vi "VariablesTCShortcutMenuCreate.vi"(8 "error in (no error)":errorcluster, 10 "ShortcutMenuIn":T2, 11 "VMUI in":refnum<class "VMUI.lvclass">) -> (0 "error out":errorcluster, 2 "Discard?":bool, 3 "VMUI out":refnum<class "VMUI.lvclass">)   [LabVIEW 2013, in "VMUI.lvclass"]
uses:
  VMUI.lvclass
  <vilib>/Utility/miscctls.llb/LVPoint32TypeDef.ctl
  VariableManager/VariableManager.lvclass
  VariableGroup/VariableGroup.lvclass
  API/VariableManagerAPI.lvlib
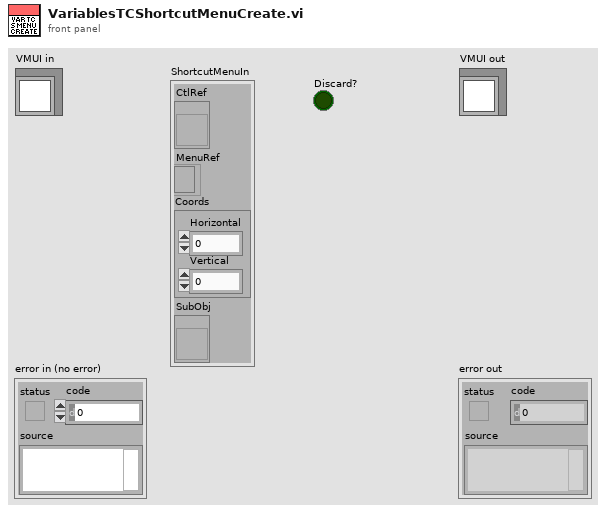
[diagram p1: front panel]
types:
  T1 = typedef "LVPoint32TypeDef.ctl" = cluster{"Horizontal":i32, "Vertical":i32}
  T2 = cluster{"CtlRef":refnum<vi>, "MenuRef":refnum<k9>, "Coords":T1, "SubObj":refnum<vi>}
  T3 = typedef "LVRowAndColumnTypeDef.ctl" = cluster{"Row":i32, "Column":i32}
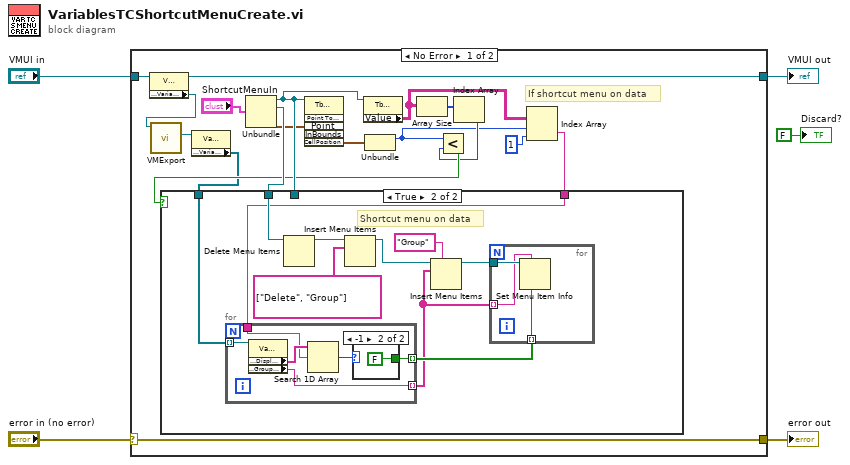
[diagram p0: block diagram]
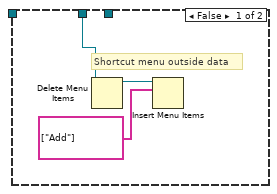
[diagram p2: hidden frame]
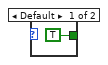
[diagram p3: hidden frame]
diagram:
  n1 = case shown="No Error" "error in (no error)" {
    selector: "error in (no error)" -> [w23 w49]
    tunnel: [w23 w49] -> w4
    tunnel: [w14 w48] -> w2
    tunnel: "VMUI in" -> [w15 w48]
    frame No Error {
      # "If shortcut menu on data"
      n2 = property class="VMUI.lvclass"(reference=w15) -> (reference out=w14:refnum<class "VMUI.lvclass">, "Accessors:VariableManagerRef"=w7:refnum<vi>)  [unwired: 1 in, 1 out]
      n3 = call "VMExport.vi"("VariableManagerRef in"=w7) -> ("VariableManagerExportCopy"=w6:refnum<class "VariableManager.lvclass">)  [unwired: 8 in, 2 out]
      n4 = property class="VariableManager.lvclass"(reference=w6) -> ("Accessors:VariableGroups"=w8:refnum<class "VariableGroup.lvclass">[])  [unwired: 1 in, 2 out]
      n5 = Unbundle("ShortcutMenuIn") -> ("CtlRef"=w22:refnum<vi>, "MenuRef"=w21:refnum<k9>, "Coords"=w16:T1)  [unwired: 1 out]
      n6 = invoke class="Tbl (strict)" method="Point To Row Column"(reference=w22, "Point"=w16) -> ("CellPosition"=w19:T3)  [unwired: 4 in, 5 out]
      n7 = property class="Tbl (strict)"(reference=w22) -> ("Value"=w13:string[][])  [unwired: 1 in, 2 out]
      n8 = Unbundle(w19) -> ("Row"=w12:i32)  [unwired: 1 out]
      n9 = Array Size(array=w13) -> (size(s)=w18:i32[])
      n10 = Index Array(array=w18) -> (element=w17:i32)  [unwired: 1 in]
      n11 = Less?(x=w12, y=w17) -> (x < y?=w20:bool)
      n12 = Index Array(array=w13, index (row)=w12, index (col)=1 ("disabled index (col)")) -> (element=w10:string)
      n13 = case shown="True" w20 {
        tunnel: w21 -> [w26 w35]
        tunnel: w22 -> [_ _]
        tunnel: w8 -> [_ w34]
        tunnel: w10 -> [_ w33]
        frame False {
          # "Shortcut menu outside data"
          n14 = Delete Menu Items(9:w26) -> (3:w25:refnum<k9>)  [unwired: 3 in, 1 out]
          n15 = Insert Menu Items(8:string[] ["Add"] ("item names"), 9:w25) -> ()  [unwired: 4 in, 3 out]
        }
        frame True {
          # "Shortcut menu on data"
          n16 = for {
            tunnel: w34 -> [w45] mode=indexing
            tunnel: w33 -> [w43]
            tunnel: [w41] -> w29 mode=indexing
            tunnel: [w40] -> w28 mode=indexing
            n17 = property class="VariableGroup.lvclass"(reference=w45) -> ("Accessors:DisplayList"=w44:string[], "Accessors:GroupName"=w40:string)  [unwired: 1 in, 2 out]
            n18 = Search 1D Array(1D array=w44, element=w43) -> (index of element=w42:i32)  [unwired: 1 in]
            n19 = case shown="-1" w42 {
              tunnel: [TRUE FALSE] -> w41
              frame Default {
              }
              frame -1 {
              }
            }
          }
          n20 = Delete Menu Items(9:w35) -> (3:w36:refnum<k9>)  [unwired: 3 in, 1 out]
          n21 = Insert Menu Items(8:string[] ["Delete", "Group"] ("item names"), 9:w36) -> (3:w32:refnum<k9>)  [unwired: 4 in, 2 out]
          n22 = Insert Menu Items(5:"Group", 8:w28, 9:w32) -> (3:w30:refnum<k9>)  [unwired: 3 in, 2 out]
          n23 = for {
            tunnel: w30 -> [w39]
            tunnel: w29 -> [w38] mode=indexing
            tunnel: w28 -> [w37] mode=indexing
            n24 = Set Menu Item Info(6:w38, 7:w37, 11:w39) -> ()  [unwired: 4 in, 2 out]
          }
        }
      }
    }
    frame Error {
    }
  }
  "error out" <- w4
  "VMUI out" <- w2
  "Discard?" <- FALSE ("Discard?")
